vi "nanocal -- nuclear schottky fit -- 2x2 -- V9.vi"() -> ()   [LabVIEW 2021] (continued)
\"mm1\" -> 0.000000000000   ,  \"mm2\" -> 0.000000000000   ,  \"mm3\" -> 0.000000000000   ,  \"T\" -> 1.120000000000   ,  \"B\" -> 10.000000000000   ,  \"θ\" -> 0.000000000000   ,  \"Reoff\" -> 0.000000000000   ,  \"Imoff\" -> 0.000000000000   ,  \"στ1\" -> 0.000000000000   ,  \"στS\" -> 0.000000000000   ,  \"στN\" -> 0.000000000000    |>   , \r\"IDS0436_220527_RAW_cal__ref_\" ->   <|    \"ζ\" -> 0.020634042480   ,  \"τ1\" -> 0.020416898580   ,  \"τS\" -> 0.013006754143   ,  \"τN\" -> 0.000157221748   ,  \"τC\" -> 0.001868338850   ,  \"κ0\" -> 0.000000012250   ,  \"mm1\" -> 0.000033184482   ,  \"mm2\" -> 0.014698009084   ,  \"mm3\" -> 0.020989645793   ,  \"T\" -> 1.900000000000   ,  \"B\" -> 10.000000000000   ,  \"θ\" -> 0.000000000000   ,  \"Reoff\" -> -693877.551020413636   ,  \"Imoff\" -> 0.000000000000   ,  \"στ1\" -> 0.001009802597   ,  \"στS\" -> 0.000108538250   ,  \"στN\" -> 0.000005592624    |>   , \r\"IDS0436_220527_RAW_cal__sam_\" ->   <|    \"ζ\" -> 0.000000000000   ,  \"τ1\" -> 0.000000000000   ,  \"τS\" -> 0.000000000000   ,  \"τN\" -> 0.000000000000   ,  \"τC\" -> 0.000000000000   ,  \"κ0\" -> 0.000000000000   ,  \"mm1\" -> 0.000000000000   ,  \"mm2\" -> 0.000000000000   ,  \"mm3\" -> 0.000000000000   ,  \"T\" -> 1.900000000000   ,  \"B\" -> 10.000000000000   ,  \"θ\" -> 0.000000000000   ,  \"Reoff\" -> 0.000000000000   ,  \"Imoff\" -> 0.000000000000   ,  \"στ1\" -> 0.000000000000   ,  \"στS\" -> 0.000000000000   ,  \"στN\" -> 0.000000000000    |>   , \r\"IDS0437_220527_RAW_cal__ref_\" ->   <|    \"ζ\" -> 0.017700486500   ,  \"τ1\" -> 0.021195716861   ,  \"τS\" -> 0.009553240691   ,  \"τN\" -> 0.000096318625   ,  \"τC\" -> 0.001777778444   ,  \"κ0\" -> 0.000000022000   ,  \"mm1\" -> 0.000026199986   ,  \"mm2\" -> 0.011360732885   ,  \"mm3\" -> 0.021406923644   ,  \"T\" -> 3.100000000000   ,  \"B\" -> 10.000000000000   ,  \"θ\" -> 0.000000000000   ,  \"Reoff\" -> -326530.612244898453   ,  \"Imoff\" -> 0.000000000000   ,  \"στ1\" -> 0.003823035587   ,  \"στS\" -> 0.000080670014   ,  \"στN\" -> 0.000008312416    |>   , \r\"IDS0437_220527_RAW_cal__sam_\" ->   <|    \"ζ\" -> 0.000000000000   ,  \"τ1\" -> 0.000000000000   ,  \"τS\" -> 0.000000000000   ,  \"τN\" -> 0.000000000000   ,  \"τC\" -> 0.000000000000   ,  \"κ0\" -> 0.000000000000   ,  \"mm1\" -> 0.000000000000   ,  \"mm2\" -> 0.000000000000   ,  \"mm3\" -> 0.000000000000   ,  \"T\" -> 3.100000000000   ,  \"B\" -> 10.000000000000   ,  \"θ\" -> 0.000000000000   ,  \"Reoff\" -> 0.000000000000   ,  \"Imoff\" -> 0.000000000000   ,  \"στ1\" -> 0.000000000000   ,  \"στS\" -> 0.000000000000   ,  \"στN\" -> 0.000000000000    |>   , \r\"IDS0438_220527_RAW_cal__ref_\" ->   <|    \"ζ\" -> 0.017333863476   ,  \"τ1\" -> 0.021487771905   ,  \"τS\" -> 0.006060943357   ,  \"τN\" -> 0.000094743973   ,  \"τC\" -> 0.001680463551   ,  \"κ0\" -> 0.000000054800   ,  \"mm1\" -> 0.000022565233   ,  \"mm2\" -> 0.007769356044   ,  \"mm3\" -> 0.021638703353   ,  \"T\" -> 5.700000000000   ,  \"B\" -> 10.000000000000   ,  \"θ\" -> 0.000000000000   ,  \"Reoff\" -> -102040.816326530650   ,  \"Imoff\" -> 0.000000000000   ,  \"στ1\" -> 0.003634760564   ,  \"στS\" -> 0.000066823566   ,  \"στN\" -> 0.000004946508    |>   , \r\"IDS0438_220527_RAW_cal__sam_\" ->   <|    \"ζ\" -> 0.000000000000   ,  \"τ1\" -> 0.000000000000   ,  \"τS\" -> 0.000000000000   ,  \"τN\" -> 0.000000000000   ,  \"τC\" -> 0.000000000000   ,  \"κ0\" -> 0.000000000000   ,  \"mm1\" -> 0.000000000000   ,  \"mm2\" -> 0.000000000000   ,  \"mm3\" -> 0.000000000000   ,  \"T\" -> 5.700000000000   ,  \"B\" -> 10.000000000000   ,  \"θ\" -> 0.000000000000   ,  \"Reoff\" -> 0.000000000000   ,  \"Imoff\" -> 0.000000000000   ,  \"στ1\" -> 0.000000000000   ,  \"στS\" -> 0.000000000000   ,  \"στN\" -> 0.000000000000    |>   , \r\"IDS0439_220527_RAW_cal__ref_\" ->   <|    \"ζ\" -> 0.020515660719   ,  \"τ1\" -> 0.020182411708   ,  \"τS\" -> 0.016419895032   ,  \"τN\" -> 0.000240616919   ,  \"τC\" -> 0.002259910162   ,  \"κ0\" -> 0.000000008010   ,  \"mm1\" -> 0.000040116981   ,  \"mm2\" -> 0.017425178232   ,  \"mm3\" -> 0.021979340018   ,  \"T\" -> 1.280000000000   ,  \"B\" -> 10.000000000000   ,  \"θ\" -> 0.000000000000   ,  \"Reoff\" -> -693877.551020413636   ,  \"Imoff\" -> 0.000000000000   ,  \"στ1\" -> 0.001720696083   ,  \"στS\" -> 0.000105898596   ,  \"στN\" -> 0.000011441558    |>   , \r\"IDS0439_220527_RAW_cal__sam_\" ->   <|    \"ζ\" -> 0.000000000000   ,  \"τ1\" -> 0.000000000000   ,  \"τS\" -> 0.000000000000   ,  \"τN\" -> 0.000000000000   ,  \"τC\" -> 0.000000000000   ,  \"κ0\" -> 0.000000000000   ,  \"mm1\" -> 0.000000000000   ,  \"mm2\" -> 0.000000000000   ,  \"mm3\" -> 0.000000000000   ,  \"T\" -> 1.280000000000   ,  \"B\" -> 10.000000000000   ,  \"θ\" -> 0.000000000000   ,  \"Reoff\" -> 0.000000000000   ,  \"Imoff\" -> 0.000000000000   ,  \"στ1\" -> 0.000000000000   ,  \"στS\" -> 0.000000000000   ,  \"στN\" -> 0.000000000000    |>   , \r\"IDS0441_220527_RAW_cal__ref_\" ->   <|    \"ζ\" -> 0.211856799532   ,  \"τ1\" -> 0.173713031248   ,  \"τS\" -> 0.025047077219   ,  \"τN\" -> 0.022799850294   ,  \"τC\" -> 0.001119487792   ,  \"κ0\" -> 0.000000000820   ,  \"mm1\" -> 0.000189887587   ,  \"mm2\" -> 0.026344768969   ,  \"mm3\" -> 0.206281486927   ,  \"T\" -> 0.200000000000   ,  \"B\" -> 6.000000000000   ,  \"θ\" -> 0.000000000000   ,  \"Reoff\" -> -7510204.081632658840   ,  \"Imoff\" -> 0.000000000000   ,  \"στ1\" -> 0.033514341427   ,  \"στS\" -> 0.000356628888   ,  \"στN\" -> 0.003953255270    |>   , \r\"IDS0441_220527_RAW_cal__sam_\" ->   <|    \"ζ\" -> 0.000000000000   ,  \"τ1\" -> 0.000000000000   ,  \"τS\" -> 0.000000000000   ,  \"τN\" -> 0.000000000000   ,  \"τC\" -> 0.000000000000   ,  \"κ0\" -> 0.000000000000   ,  \"mm1\" -> 0.000000000000   ,  \"mm2\" -> 0.000000000000   ,  \"mm3\" -> 0.000000000000   ,  \"T\" -> 0.200000000000   ,  \"B\" -> 6.000000000000   ,  \"θ\" -> 0.000000000000   ,  \"Reoff\" -> 0.000000000000   ,  \"Imoff\" -> 0.000000000000   ,  \"στ1\" -> 0.000000000000   ,  \"στS\" -> 0.000000000000   ,  \"στN\" -> 0.000000000000    |>   , \r\"IDS0442_220528_RAW_cal__ref_\" ->   <|    \"ζ\" -> 0.627289985820   ,  \"τ1\" -> 0.239743496780   ,  \"τS\" -> 0.076926495749   ,  \"τN\" -> 0.159415903746   ,  \"τC\" -> 0.000763641667   ,  \"κ0\" -> 0.000000000435   ,  \"mm1\" -> 0.000293264880   ,  \"mm2\" -> 0.052650493650   ,  \"mm3\" -> 0.572160999840   ,  \"T\" -> 0.120000000000   ,  \"B\" -> 6.000000000000   ,  \"θ\" -> 0.000000000000   ,  \"Reoff\" -> -187755102.040816367000   ,  \"Imoff\" -> 0.000000000000   ,  \"στ1\" -> 0.245568364347   ,  \"στS\" -> 0.022170590915   ,  \"στN\" -> 0.126655465898    |>   , \r\"IDS0442_220528_RAW_cal__sam_\" ->   <|    \"ζ\" -> 0.000000000000   ,  \"τ1\" -> 0.000000000000   ,  \"τS\" -> 0.000000000000   ,  \"τN\" -> 0.000000000000   ,  \"τC\" -> 0.000000000000   ,  \"κ0\" -> 0.000000000000   ,  \"mm1\" -> 0.000000000000   ,  \"mm2\" -> 0.000000000000   ,  \"mm3\" -> 0.000000000000   ,  \"T\" -> 0.120000000000   ,  \"B\" -> 6.000000000000   ,  \"θ\" -> 0.000000000000   ,  \"Reoff\" -> 0.000000000000   ,  \"Imoff\" -> 0.000000000000   ,  \"στ1\" -> 0.000000000000   ,  \"στS\" -> 0.000000000000   ,  \"στN\" -> 0.000000000000    |>   , \r\"IDS0443_220528_RAW_cal__ref_\" ->   <|    \"ζ\" -> 0.436035823116   ,  \"τ1\" -> 0.136298324856   ,  \"τS\" -> 0.035428802447   ,  \"τN\" -> 0.042141009445   ,  \"τC\" -> 0.000863434496   ,  \"κ0\" -> 0.000000000631   ,  \"mm1\" -> 0.000259087412   ,  \"mm2\" -> 0.032519927017   ,  \"mm3\" -> 0.215775773592   ,  \"T\" -> 0.150000000000   ,  \"B\" -> 6.000000000000   ,  \"θ\" -> 0.000000000000   ,  \"Reoff\" -> -60040816.326530613000   ,  \"Imoff\" -> 0.000000000000   ,  \"στ1\" -> 0.080047050506   ,  \"στS\" -> 0.002312030387   ,  \"στN\" -> 0.019370507574    |>   , \r\"IDS0443_220528_RAW_cal__sam_\" ->   <|    \"ζ\" -> 0.000000000000   ,  \"τ1\" -> 0.000000000000   ,  \"τS\" -> 0.000000000000   ,  \"τN\" -> 0.000000000000   ,  \"τC\" -> 0.000000000000   ,  \"κ0\" -> 0.000000000000   ,  \"mm1\" -> 0.000000000000   ,  \"mm2\" -> 0.000000000000   ,  \"mm3\" -> 0.000000000000   ,  \"T\" -> 0.150000000000   ,  \"B\" -> 6.000000000000   ,  \"θ\" -> 0.000000000000   ,  \"Reoff\" -> 0.000000000000   ,  \"Imoff\" -> 0.000000000000   ,  \"στ1\" -> 0.000000000000   ,  \"στS\" -> 0.000000000000   ,  \"στN\" -> 0.000000000000    |>   , \r\"IDS0444_220528_RAW_cal__ref_\" ->   <|    \"ζ\" -> 0.312738827075   ,  \"τ1\" -> 0.153166775684   ,  \"τS\" -> 0.029428403772   ,  \"τN\" -> 0.032059842595   ,  \"τC\" -> 0.000966119229   ,  \"κ0\" -> 0.000000000763   ,  \"mm1\" -> 0.000225827852   ,  \"mm2\" -> 0.029383297615   ,  \"mm3\" -> 0.205241777861   ,  \"T\" -> 0.170000000000   ,  \"B\" -> 6.000000000000   ,  \"θ\" -> 0.000000000000   ,  \"Reoff\" -> -20979591.836734697200   ,  \"Imoff\" -> 0.000000000000   ,  \"στ1\" -> 0.194871487206   ,  \"στS\" -> 0.001481931895   ,  \"στN\" -> 0.032515587695    |>   , \r\"IDS0444_220528_RAW_cal__sam_\" ->   <|    \"ζ\" -> 0.000000000000   ,  \"τ1\" -> 0.000000000000   ,  \"τS\" -> 0.000000000000   ,  \"τN\" -> 0.000000000000   ,  \"τC\" -> 0.000000000000   ,  \"κ0\" -> 0.000000000000   ,  \"mm1\" -> 0.000000000000   ,  \"mm2\" -> 0.000000000000   ,  \"mm3\" -> 0.000000000000   ,  \"T\" -> 0.170000000000   ,  \"B\" -> 6.000000000000   ,  \"θ\" -> 0.000000000000   ,  \"Reoff\" -> 0.000000000000   ,  \"Imoff\" -> 0.000000000000   ,  \"στ1\" -> 0.000000000000   ,  \"στS\" -> 0.000000000000   ,  \"στN\" -> 0.000000000000    |>   , \r\"IDS0445_220528_RAW_cal__ref_\" ->   <|    \"ζ\" -> 0.144974292956   ,  \"τ1\" -> 0.278153679109   ,  \"τS\" -> 0.020087180736   ,  \"τN\" -> 0.018878235169   ,  \"τC\" -> 0.001360650262   ,  \"κ0\" -> 0.000000001251   ,  \"mm1\" -> 0.000163756081   ,  \"mm2\" -> 0.022311875645   ,  \"mm3\" -> 0.301653097172   ,  \"T\" -> 0.250000000000   ,  \"B\" -> 6.000000000000   ,  \"θ\" -> 0.000000000000   ,  \"Reoff\" -> -857142.857142856343   ,  \"Imoff\" -> 0.000000000000   ,  \"στ1\" -> 0.021844314170   ,  \"στS\" -> 0.000158941721   ,  \"στN\" -> 0.001374609128    |>   , \r\"IDS0445_220528_RAW_cal__sam_\" ->   <|    \"ζ\" -> 0.000000000000   ,  \"τ1\" -> 0.000000000000   ,  \"τS\" -> 0.000000000000   ,  \"τN\" -> 0.000000000000   ,  \"τC\" -> 0.000000000000   ,  \"κ0\" -> 0.000000000000   ,  \"mm1\" -> 0.000000000000   ,  \"mm2\" -> 0.000000000000   ,  \"mm3\" -> 0.000000000000   ,  \"T\" -> 0.250000000000   ,  \"B\" -> 6.000000000000   ,  \"θ\" -> 0.000000000000   ,  \"Reoff\" -> 0.000000000000   ,  \"Imoff\" -> 0.000000000000   ,  \"στ1\" -> 0.000000000000   ,  \"στS\" -> 0.000000000000   ,  \"στN\" -> 0.000000000000    |>   , \r\"IDS0446_220528_RAW_cal__ref_\" ->   <|    \"ζ\" -> 0.103205072553   ,  \"τ1\" -> 0.456877167810   ,  \"τS\" -> 0.018190810680   ,  \"τN\" -> 0.020353539569   ,  \"τC\" -> 0.001532633678   ,  \"κ0\" -> 0.000000001557   ,  \"mm1\" -> 0.000134033999   ,  \"mm2\" -> 0.020416907251   ,  \"mm3\" -> 0.480381182951   ,  \"T\" -> 0.300000000000   ,  \"B\" -> 6.000000000000   ,  \"θ\" -> 0.000000000000   ,  \"Reoff\" -> -461224.489795918343   ,  \"Imoff\" -> 0.000000000000   ,  \"στ1\" -> 0.032347659490   ,  \"στS\" -> 0.000102258041   ,  \"στN\" -> 0.001172701872    |>   , \r\"IDS0446_220528_RAW_cal__sam_\" ->   <|    \"ζ\" -> 0.000000000000   ,  \"τ1\" -> 0.000000000000   ,  \"τS\" -> 0.000000000000   ,  \"τN\" -> 0.000000000000   ,  \"τC\" -> 0.000000000000   ,  \"κ0\" -> 0.000000000000   ,  \"mm1\" -> 0.000000000000   ,  \"mm2\" -> 0.000000000000   ,  \"mm3\" -> 0.000000000000   ,  \"T\" -> 0.300000000000   ,  \"B\" -> 6.000000000000   ,  \"θ\" -> 0.000000000000   ,  \"Reoff\" -> 0.000000000000   ,  \"Imoff\" -> 0.000000000000   ,  \"στ1\" -> 0.000000000000   ,  \"στS\" -> 0.000000000000   ,  \"στN\" -> 0.000000000000    |>   , \r\"IDS0447_220528_RAW_cal__ref_\" ->   <|    \"ζ\" -> 0.067386498273   ,  \"τ1\" -> 0.033759383158   ,  \"τS\" -> 0.016352467508   ,  \"τN\" -> 0.000055602042   ,  \"τC\" -> 0.002052818742   ,  \"κ0\" -> 0.000000002053   ,  \"mm1\" -> 0.000116658355   ,  \"mm2\" -> 0.019311291178   ,  \"mm3\" -> 0.033898004267   ,  \"T\" -> 0.360000000000   ,  \"B\" -> 6.000000000000   ,  \"θ\" -> 0.000000000000   ,  \"Reoff\" -> 4122448.979591837150   ,  \"Imoff\" -> 0.000000000000   ,  \"στ1\" -> 0.002480419110   ,  \"στS\" -> 0.000128292028   ,  \"στN\" -> 0.000001339614    |>   , \r\"IDS0447_220528_RAW_cal__sam_\" ->   <|    \"ζ\" -> 0.000000000000   ,  \"τ1\" -> 0.000000000000   ,  \"τS\" -> 0.000000000000   ,  \"τN\" -> 0.000000000000   ,  \"τC\" -> 0.000000000000   ,  \"κ0\" -> 0.000000000000   ,  \"mm1\" -> 0.000000000000   ,  \"mm2\" -> 0.000000000000   ,  \"mm3\" -> 0.000000000000   ,  \"T\" -> 0.360000000000   ,  \"B\" -> 6.000000000000   ,  \"θ\" -> 0.000000000000   ,  \"Reoff\" -> 0.000000000000   ,  \"Imoff\" -> 0.000000000000   ,  \"στ1\" -> 0.000000000000   ,  \"στS\" -> 0.000000000000   ,  \"στN\" -> 0.000000000000    |>   , \r\"IDS0448_220528_RAW_cal__ref_\" ->   <|    \"ζ\" -> 0.022507492936   ,  \"τ1\" -> 0.033871434243   ,  \"τS\" -> 0.016835987173   ,  \"τN\" -> 0.000213468402   ,  \"τC\" -> 0.001778165835   ,  \"κ0\" -> 0.000000002480   ,  \"mm1\" -> 0.000035543102   ,  \"mm2\" -> 0.018688914469   ,  \"mm3\" -> 0.034358338584   ,  \"T\" -> 0.420000000000   ,  \"B\" -> 6.000000000000   ,  \"θ\" -> 0.000000000000   ,  \"Reoff\" -> 4122448.979591837150   ,  \"Imoff\" -> 0.000000000000   ,  \"στ1\" -> 0.007814821926   ,  \"στS\" -> 0.000385740474   ,  \"στN\" -> 0.000018309382    |>   , \r\"IDS0448_220528_RAW_cal__sam_\" ->   <|    \"ζ\" -> 0.000000000000   ,  \"τ1\" -> 0.000000000000   ,  \"τS\" -> 0.000000000000   ,  \"τN\" -> 0.000000000000   ,  \"τC\" -> 0.000000000000   ,  \"κ0\" -> 0.000000000000   ,  \"mm1\" -> 0.000000000000   ,  \"mm2\" -> 0.000000000000   ,  \"mm3\" -> 0.000000000000   ,  \"T\" -> 0.420000000000   ,  \"B\" -> 6.000000000000   ,  \"θ\" -> 0.000000000000   ,  \"Reoff\" -> 0.000000000000   ,  \"Imoff\" -> 0.000000000000   ,  \"στ1\" -> 0.000000000000   ,  \"στS\" -> 0.000000000000   ,  \"στN\" -> 0.000000000000    |>   , \r\"IDS0449_220528_RAW_cal__ref_\" ->   <|    \"ζ\" -> 0.021849716435   ,  \"τ1\" -> 0.033883152649   ,  \"τS\" -> 0.018197027738   ,  \"τN\" -> 0.000213402501   ,  \"τC\" -> 0.001801850307   ,  \"κ0\" -> 0.000000003131   ,  \"mm1\" -> 0.000035185130   ,  \"mm2\" -> 0.020045453610   ,  \"mm3\" -> 0.034417057136   ,  \"T\" -> 0.520000000000   ,  \"B\" -> 6.000000000000   ,  \"θ\" -> 0.000000000000   ,  \"Reoff\" -> 4122448.979591837150   ,  \"Imoff\" -> 0.000000000000   ,  \"στ1\" -> 0.005200135882   ,  \"στS\" -> 0.000196781752   ,  \"στN\" -> 0.000016694885    |>   , \r\"IDS0449_220528_RAW_cal__sam_\" ->   <|    \"ζ\" -> 0.000000000000   ,  \"τ1\" -> 0.000000000000   ,  \"τS\" -> 0.000000000000   ,  \"τN\" -> 0.000000000000   ,  \"τC\" -> 0.000000000000   ,  \"κ0\" -> 0.000000000000   ,  \"mm1\" -> 0.000000000000   ,  \"mm2\" -> 0.000000000000   ,  \"mm3\" -> 0.000000000000   ,  \"T\" -> 0.520000000000   ,  \"B\" -> 6.000000000000   ,  \"θ\" -> 0.000000000000   ,  \"Reoff\" -> 0.000000000000   ,  \"Imoff\" -> 0.000000000000   ,  \"στ1\" -> 0.000000000000   ,  \"στS\" -> 0.000000000000   ,  \"στN\" -> 0.000000000000    |>   , \r\"IDS0450_220528_RAW_cal__ref_\" ->   <|    \"ζ\" -> 0.021729475893   ,  \"τ1\" -> 0.033901786343   ,  \"τS\" -> 0.020153498516   ,  \"τN\" -> 0.000213217921   ,  \"τC\" -> 0.001808973424   ,  \"κ0\" -> 0.000000003806   ,  \"mm1\" -> 0.000035421184   ,  \"mm2\" -> 0.021964202896   ,  \"mm3\" -> 0.034520410198   ,  \"T\" -> 0.620000000000   ,  \"B\" -> 6.000000000000   ,  \"θ\" -> 0.000000000000   ,  \"Reoff\" -> 3061224.489795919510   ,  \"Imoff\" -> 0.000000000000   ,  \"στ1\" -> 0.006296094438   ,  \"στS\" -> 0.000269248074   ,  \"στN\" -> 0.000016264647    |>   , \r\"IDS0450_220528_RAW_cal__sam_\" ->   <|    \"ζ\" -> 0.000000000000   ,  \"τ1\" -> 0.000000000000   ,  \"τS\" -> 0.000000000000   ,  \"τN\" -> 0.000000000000   ,  \"τC\" -> 0.000000000000   ,  \"κ0\" -> 0.000000000000   ,  \"mm1\" -> 0.000000000000   ,  \"mm2\" -> 0.000000000000   ,  \"mm3\" -> 0.000000000000   ,  \"T\" -> 0.620000000000   ,  \"B\" -> 6.000000000000   ,  \"θ\" -> 0.000000000000   ,  \"Reoff\" -> 0.000000000000   ,  \"Imoff\" -> 0.000000000000   ,  \"στ1\" -> 0.000000000000   ,  \"στS\" -> 0.000000000000   ,  \"στN\" -> 0.000000000000    |>   , \r\"IDS0451_220528_RAW_cal__ref_\" ->   <|    \"ζ\" -> 0.019851972634   ,  \"τ1\" -> 0.033846561532   ,  \"τS\" -> 0.023547995636   ,  \"τN\" -> 0.000274131753   ,  \"τC\" -> 0.002984103948   ,  \"κ0\" -> 0.000000005214   ,  \"mm1\" -> 0.000051766319   ,  \"mm2\" -> 0.026018760545   ,  \"mm3\" -> 0.035055182225   ,  \"T\" -> 0.820000000000   ,  \"B\" -> 6.000000000000   ,  \"θ\" -> 0.000000000000   ,  \"Reoff\" -> 40816.326530613005   ,  \"Imoff\" -> 0.000000000000   ,  \"στ1\" -> 0.001908169809   ,  \"στS\" -> 0.000133930876   ,  \"στN\" -> 0.000002638452    |>   , \r\"IDS0451_220528_RAW_cal__sam_\" ->   <|    \"ζ\" -> 0.000000000000   ,  \"τ1\" -> 0.000000000000   ,  \"τS\" -> 0.000000000000   ,  \"τN\" -> 0.000000000000   ,  \"τC\" -> 0.000000000000   ,  \"κ0\" -> 0.000000000000   ,  \"mm1\" -> 0.000000000000   ,  \"mm2\" -> 0.000000000000   ,  \"mm3\" -> 0.000000000000   ,  \"T\" -> 0.820000000000   ,  \"B\" -> 6.000000000000   ,  \"θ\" -> 0.000000000000   ,  \"Reoff\" -> 0.000000000000   ,  \"Imoff\" -> 0.000000000000   ,  \"στ1\" -> 0.000000000000   ,  \"στS\" -> 0.000000000000   ,  \"στN\" -> 0.000000000000    |>   , \r\"IDS0452_220528_RAW_cal__ref_\" ->   <|    \"ζ\" -> 0.016283381951   ,  \"τ1\" -> 0.033904524460   ,  \"τS\" -> 0.031661688913   ,  \"τN\" -> 0.000274537016   ,  \"τC\" -> 0.003250738485   ,  \"κ0\" -> 0.000000007263   ,  \"mm1\" -> 0.000047369067   ,  \"mm2\" -> 0.031583889293   ,  \"mm3\" -> 0.037980260279   ,  \"T\" -> 1.120000000000   ,  \"B\" -> 6.000000000000   ,  \"θ\" -> 0.000000000000   ,  \"Reoff\" -> 40816.326530613005   ,  \"Imoff\" -> 0.000000000000   ,  \"στ1\" -> 0.002257620140   ,  \"στS\" -> 0.000162839807   ,  \"στN\" -> 0.000009699550    |>   , \r\"IDS0452_220528_RAW_cal__sam_\" ->   <|    \"ζ\" -> 0.000000000000   ,  \"τ1\" -> 0.000000000000   ,  \"τS\" -> 0.000000000000   ,  \"τN\" -> 0.000000000000   ,  \"τC\" -> 0.000000000000   ,  \"κ0\" -> 0.000000000000   ,  \"mm1\" -> 0.000000000000   ,  \"mm2\" -> 0.000000000000   ,  \"mm3\" -> 0.000000000000   ,  \"T\" -> 1.120000000000   ,  \"B\" -> 6.000000000000   ,  \"θ\" -> 0.000000000000   ,  \"Reoff\" -> 0.000000000000   ,  \"Imoff\" -> 0.000000000000   ,  \"στ1\" -> 0.000000000000   ,  \"στS\" -> 0.000000000000   ,  \"στN\" -> 0.000000000000    |>   , \r\"IDS0453_220529_RAW_cal__ref_\" ->   <|    \"ζ\" -> 0.018860897000   ,  \"τ1\" -> 0.033783692310   ,  \"τS\" -> 0.033495916545   ,  \"τN\" -> 0.000426157498   ,  \"τC\" -> 0.003160296043   ,  \"κ0\" -> 0.000000011406   ,  \"mm1\" -> 0.000053621310   ,  \"mm2\" -> 0.031431982647   ,  \"mm3\" -> 0.040020259184   ,  \"T\" -> 1.700000000000   ,  \"B\" -> 6.000000000000   ,  \"θ\" -> 0.000000000000   ,  \"Reoff\" -> -371428.571428571827   ,  \"Imoff\" -> 0.000000000000   ,  \"στ1\" -> 0.008605835969   ,  \"στS\" -> 0.000457782614   ,  \"στN\" -> 0.000070271904    |>   , \r\"IDS0453_220529_RAW_cal__sam_\" ->   <|    \"ζ\" -> 0.000000000000   ,  \"τ1\" -> 0.000000000000   ,  \"τS\" -> 0.000000000000   ,  \"τN\" -> 0.000000000000   ,  \"τC\" -> 0.000000000000   ,  \"κ0\" -> 0.000000000000   ,  \"mm1\" -> 0.000000000000   ,  \"mm2\" -> 0.000000000000   ,  \"mm3\" -> 0.000000000000   ,  \"T\" -> 1.700000000000   ,  \"B\" -> 6.000000000000   ,  \"θ\" -> 0.000000000000   ,  \"Reoff\" -> 0.000000000000   ,  \"Imoff\" -> 0.000000000000   ,  \"στ1\" -> 0.000000000000   ,  \"στS\" -> 0.000000000000   ,  \"στN\" -> 0.000000000000    |>   , \r\"IDS0454_220529_RAW_cal__ref_\" ->   <|    \"ζ\" -> 0.017534515106   ,  \"τ1\" -> 0.023238617838   ,  \"τS\" -> 0.014265591932   ,  \"τN\" -> 0.000383027801   ,  \"τC\" -> 0.002949269667   ,  \"κ0\" -> 0.000000012895   ,  \"mm1\" -> 0.000042342847   ,  \"mm2\" -> 0.016473998003   ,  \"mm3\" -> 0.024577022833   ,  \"T\" -> 1.900000000000   ,  \"B\" -> 6.000000000000   ,  \"θ\" -> 0.000000000000   ,  \"Reoff\" -> -371428.571428571827   ,  \"Imoff\" -> 0.000000000000   ,  \"στ1\" -> 0.002498996258   ,  \"στS\" -> 0.000312031837   ,  \"στN\" -> 0.000009499626    |>   , \r\"IDS0454_220529_RAW_cal__sam_\" ->   <|    \"ζ\" -> 0.000000000000   ,  \"τ1\" -> 0.000000000000   ,  \"τS\" -> 0.000000000000   ,  \"τN\" -> 0.000000000000   ,  \"τC\" -> 0.000000000000   ,  \"κ0\" -> 0.000000000000   ,  \"mm1\" -> 0.000000000000   ,  \"mm2\" -> 0.000000000000   ,  \"mm3\" -> 0.000000000000   ,  \"T\" -> 1.900000000000   ,  \"B\" -> 6.000000000000   ,  \"θ\" -> 0.000000000000   ,  \"Reoff\" -> 0.000000000000   ,  \"Imoff\" -> 0.000000000000   ,  \"στ1\" -> 0.000000000000   ,  \"στS\" -> 0.000000000000   ,  \"στN\" -> 0.000000000000    |>   , \r\"IDS0455_220529_RAW_cal__ref_\" ->   <|    \"ζ\" -> 0.016579016475   ,  \"τ1\" -> 0.029207680039   ,  \"τS\" -> 0.009191722708   ,  \"τN\" -> 0.000282214156   ,  \"τC\" -> 0.002421267657   ,  \"κ0\" -> 0.000000022277   ,  \"mm1\" -> 0.000031445020   ,  \"mm2\" -> 0.011546501346   ,  \"mm3\" -> 0.029682006750   ,  \"T\" -> 3.100000000000   ,  \"B\" -> 6.000000000000   ,  \"θ\" -> 0.000000000000   ,  \"Reoff\" -> -224489.795918366871   ,  \"Imoff\" -> 0.000000000000   ,  \"στ1\" -> 0.003215464239   ,  \"στS\" -> 0.000088801730   ,  \"στN\" -> 0.000015299267    |>   , \r\"IDS0455_220529_RAW_cal__sam_\" ->   <|    \"ζ\" -> 0.000000000000   ,  \"τ1\" -> 0.000000000000   ,  \"τS\" -> 0.000000000000   ,  \"τN\" -> 0.000000000000   ,  \"τC\" -> 0.000000000000   ,  \"κ0\" -> 0.000000000000   ,  \"mm1\" -> 0.000000000000   ,  \"mm2\" -> 0.000000000000   ,  \"mm3\" -> 0.000000000000   ,  \"T\" -> 3.100000000000   ,  \"B\" -> 6.000000000000   ,  \"θ\" -> 0.000000000000   ,  \"Reoff\" -> 0.000000000000   ,  \"Imoff\" -> 0.000000000000   ,  \"στ1\" -> 0.000000000000   ,  \"στS\" -> 0.000000000000   ,  \"στN\" -> 0.000000000000    |>   , \r\"IDS0456_220529_RAW_cal__ref_\" ->   <|    \"ζ\" -> 0.017491792324   ,  \"τ1\" -> 0.025875515293   ,  \"τS\" -> 0.005854448604   ,  \"τN\" -> 0.000336782612   ,  \"τC\" -> 0.002022629565   ,  \"κ0\" -> 0.000000054778   ,  \"mm1\" -> 0.000026042057   ,  \"mm2\" -> 0.007805583534   ,  \"mm3\" -> 0.026366046213   ,  \"T\" -> 5.700000000000   ,  \"B\" -> 6.000000000000   ,  \"θ\" -> 0.000000000000   ,  \"Reoff\" -> -77551.020408162847   ,  \"Imoff\" -> 0.000000000000   ,  \"στ1\" -> 0.003570816055   ,  \"στS\" -> 0.000072912365   ,  \"στN\" -> 0.000023576375    |>   , \r\"IDS0456_220529_RAW_cal__sam_\" ->   <|    \"ζ\" -> 0.000000000000   ,  \"τ1\" -> 0.000000000000   ,  \"τS\" -> 0.000000000000   ,  \"τN\" -> 0.000000000000   ,  \"τC\" -> 0.000000000000   ,  \"κ0\" -> 0.000000000000   ,  \"mm1\" -> 0.000000000000   ,  \"mm2\" -> 0.000000000000   ,  \"mm3\" -> 0.000000000000   ,  \"T\" -> 5.700000000000   ,  \"B\" -> 6.000000000000   ,  \"θ\" -> 0.000000000000   ,  \"Reoff\" -> 0.000000000000   ,  \"Imoff\" -> 0.000000000000   ,  \"στ1\" -> 0.000000000000   ,  \"στS\" -> 0.000000000000   ,  \"στN\" -> 0.000000000000    |>   , \r\"IDS0458_220529_RAW_cal__ref_\" ->   <|    \"ζ\" -> 0.258233838884   ,  \"τ1\" -> 0.194823836197   ,  \"τS\" -> 0.017297068774   ,  \"τN\" -> 0.011336600616   ,  \"τC\" -> 0.000861022284   ,  \"κ0\" -> 0.000000000878   ,  \"mm1\" -> 0.000171280662   ,  \"mm2\" -> 0.020753326511   ,  \"mm3\" -> 0.210788103067   ,  \"T\" -> 0.200000000000   ,  \"B\" -> 4.000000000000   ,  \"θ\" -> 0.000000000000   ,  \"Reoff\" -> -40000000.000000000000   ,  \"Imoff\" -> 0.000000000000   ,  \"στ1\" -> 0.011784060995   ,  \"στS\" -> 0.000101210120   ,  \"στN\" -> 0.000651260820    |>   , \r\"IDS0458_220529_RAW_cal__sam_\" ->   <|    \"ζ\" -> 0.000000000000   ,  \"τ1\" -> 0.000000000000   ,  \"τS\" -> 0.000000000000   ,  \"τN\" -> 0.000000000000   ,  \"τC\" -> 0.000000000000   ,  \"κ0\" -> 0.000000000000   ,  \"mm1\" -> 0.000000000000   ,  \"mm2\" -> 0.000000000000   ,  \"mm3\" -> 0.000000000000   ,  \"T\" -> 0.200000000000   ,  \"B\" -> 4.000000000000   ,  \"θ\" -> 0.000000000000   ,  \"Reoff\" -> 0.000000000000   ,  \"Imoff\" -> 0.000000000000   ,  \"στ1\" -> 0.000000000000   ,  \"στS\" -> 0.000000000000   ,  \"στN\" -> 0.000000000000    |>   , \r\"IDS0459_220529_RAW_cal__ref_\" ->   <|    \"ζ\" -> 0.141553441331   ,  \"τ1\" -> 0.275028685548   ,  \"τS\" -> 0.015047963076   ,  \"τN\" -> 0.008277224775   ,  \"τC\" -> 0.000952592092   ,  \"κ0\" -> 0.000000001241   ,  \"mm1\" -> 0.000112614213   ,  \"mm2\" -> 0.017380815596   ,  \"mm3\" -> 0.285114796291   ,  \"T\" -> 0.250000000000   ,  \"B\" -> 4.000000000000   ,  \"θ\" -> 0.000000000000   ,  \"Reoff\" -> -3469387.755102038380   ,  \"Imoff\" -> 0.000000000000   ,  \"στ1\" -> 0.080083912968   ,  \"στS\" -> 0.000323805497   ,  \"στN\" -> 0.002416154276    |>   , \r\"IDS0459_220529_RAW_cal__sam_\" ->   <|    \"ζ\" -> 0.000000000000   ,  \"τ1\" -> 0.000000000000   ,  \"τS\" -> 0.000000000000   ,  \"τN\" -> 0.000000000000   ,  \"τC\" -> 0.000000000000   ,  \"κ0\" -> 0.000000000000   ,  \"mm1\" -> 0.000000000000   ,  \"mm2\" -> 0.000000000000   ,  \"mm3\" -> 0.000000000000   ,  \"T\" -> 0.250000000000   ,  \"B\" -> 4.000000000000   ,  \"θ\" -> 0.000000000000   ,  \"Reoff\" -> 0.000000000000   ,  \"Imoff\" -> 0.000000000000   ,  \"στ1\" -> 0.000000000000   ,  \"στS\" -> 0.000000000000   ,  \"στN\" -> 0.000000000000    |>   , \r\"IDS0460_220529_RAW_cal__ref_\" ->   <|    \"ζ\" -> 0.100306525535   ,  \"τ1\" -> 0.323446583464   ,  \"τS\" -> 0.014112138770   ,  \"τN\" -> 0.006689862663   ,  \"τC\" -> 0.001003931407   ,  \"κ0\" -> 0.000000001578   ,  \"mm1\" -> 0.000086413968   ,  \"mm2\" -> 0.016060715827   ,  \"mm3\" -> 0.331191962998   ,  \"T\" -> 0.300000000000   ,  \"B\" -> 4.000000000000   ,  \"θ\" -> 0.000000000000   ,  \"Reoff\" -> -1346938.775510203090   ,  \"Imoff\" -> 0.000000000000   ,  \"στ1\" -> 0.228013917636   ,  \"στS\" -> 0.000228957843   ,  \"στN\" -> 0.004274163524    |>   , \r\"IDS0460_220529_RAW_cal__sam_\" ->   <|    \"ζ\" -> 0.000000000000   ,  \"τ1\" -> 0.000000000000   ,  \"τS\" -> 0.000000000000   ,  \"τN\" -> 0.000000000000   ,  \"τC\" -> 0.000000000000   ,  \"κ0\" -> 0.000000000000   ,  \"mm1\" -> 0.000000000000   ,  \"mm2\" -> 0.000000000000   ,  \"mm3\" -> 0.000000000000   ,  \"T\" -> 0.300000000000   ,  \"B\" -> 4.000000000000   ,  \"θ\" -> 0.000000000000   ,  \"Reoff\" -> 0.000000000000   ,  \"Imoff\" -> 0.000000000000   ,  \"στ1\" -> 0.000000000000   ,  \"στS\" -> 0.000000000000   ,  \"στN\" -> 0.000000000000    |>   , \r\"IDS0461_220529_RAW_cal__ref_\" ->   <|    \"ζ\" -> 0.071863540355   ,  \"τ1\" -> 0.372398952116   ,  \"τS\" -> 0.013146723142   ,  \"τN\" -> 0.005489502105   ,  \"τC\" -> 0.001555491237   ,  \"κ0\" -> 0.000000001966   ,  \"mm1\" -> 0.000094490759   ,  \"mm2\" -> 0.015300544387   ,  \"mm3\" -> 0.378534898581   ,  \"T\" -> 0.360000000000   ,  \"B\" -> 4.000000000000   ,  \"θ\" -> 0.000000000000   ,  \"Reoff\" -> 40816.326530613005   ,  \"Imoff\" -> 0.000000000000   ,  \"στ1\" -> 0.066981077453   ,  \"στS\" -> 0.000100786284   ,  \"στN\" -> 0.000881671068    |>   , \r\"IDS0461_220529_RAW_cal__sam_\" ->   <|    \"ζ\" -> 0.000000000000   ,  \"τ1\" -> 0.000000000000   ,  \"τS\" -> 0.000000000000   ,  \"τN\" -> 0.000000000000   ,  \"τC\" -> 0.000000000000   ,  \"κ0\" -> 0.000000000000   ,  \"mm1\" -> 0.000000000000   ,  \"mm2\" -> 0.000000000000   ,  \"mm3\" -> 0.000000000000   ,  \"T\" -> 0.360000000000   ,  \"B\" -> 4.000000000000   ,  \"θ\" -> 0.000000000000   ,  \"Reoff\" -> 0.000000000000   ,  \"Imoff\" -> 0.000000000000   ,  \"στ1\" -> 0.000000000000   ,  \"στS\" -> 0.000000000000   ,  \"στN\" -> 0.000000000000    |>   , \r\"IDS0462_220530_RAW_cal__ref_\" ->   <|    \"ζ\" -> 0.346375365864   ,  \"τ1\" -> 0.255981907492   ,  \"τS\" -> 0.020113199989   ,  \"τN\" -> 0.019024971264   ,  \"τC\" -> 0.000835805308   ,  \"κ0\" -> 0.000000000713   ,  \"mm1\" -> 0.000210164212   ,  \"mm2\" -> 0.024940973157   ,  \"mm3\" -> 0.284361245071   ,  \"T\" -> 0.170000000000   ,  \"B\" -> 4.000000000000   ,  \"θ\" -> 0.000000000000   ,  \"Reoff\" -> -62857142.857142865700   ,  \"Imoff\" -> 0.000000000000   ,  \"στ1\" -> 0.079526914499   ,  \"στS\" -> 0.000288042615   ,  \"στN\" -> 0.004319163627    |>   , \r\"IDS0462_220530_RAW_cal__sam_\" ->   <|    \"ζ\" -> 0.000000000000   ,  \"τ1\" -> 0.000000000000   ,  \"τS\" -> 0.000000000000   ,  \"τN\" -> 0.000000000000   ,  \"τC\" -> 0.000000000000   ,  \"κ0\" -> 0.000000000000   ,  \"mm1\" -> 0.000000000000   ,  \"mm2\" -> 0.000000000000   ,  \"mm3\" -> 0.000000000000   ,  \"T\" -> 0.170000000000   ,  \"B\" -> 4.000000000000   ,  \"θ\" -> 0.000000000000   ,  \"Reoff\" -> 0.000000000000   ,  \"Imoff\" -> 0.000000000000   ,  \"στ1\" -> 0.000000000000   ,  \"στS\" -> 0.000000000000   ,  \"στN\" -> 0.000000000000    |>   , \r\"IDS0463_220530_RAW_cal__ref_\" ->   <|    \"ζ\" -> 0.446275337285   ,  \"τ1\" -> 0.266780954732   ,  \"τS\" -> 0.022382001002   ,  \"τN\" -> 0.026082260900   ,  \"τC\" -> 0.000765140515   ,  \"κ0\" -> 0.000000000610   ,  \"mm1\" -> 0.000232271004   ,  \"mm2\" -> 0.028408418126   ,  \"mm3\" -> 0.308998072845   ,  \"T\" -> 0.150000000000   ,  \"B\" -> 4.000000000000   ,  \"θ\" -> 0.000000000000   ,  \"Reoff\" -> -99591836.734693884900   ,  \"Imoff\" -> 0.000000000000   ,  \"στ1\" -> 0.224882550084   ,  \"στS\" -> 0.000618191534   ,  \"στN\" -> 0.017485695172    |>   , \r\"IDS0463_220530_RAW_cal__sam_\" ->   <|    \"ζ\" -> 0.000000000000   ,  \"τ1\" -> 0.000000000000   ,  \"τS\" -> 0.000000000000   ,  \"τN\" -> 0.000000000000   ,  \"τC\" -> 0.000000000000   ,  \"κ0\" -> 0.000000000000   ,  \"mm1\" -> 0.000000000000   ,  \"mm2\" -> 0.000000000000   ,  \"mm3\" -> 0.000000000000   ,  \"T\" -> 0.150000000000   ,  \"B\" -> 4.000000000000   ,  \"θ\" -> 0.000000000000   ,  \"Reoff\" -> 0.000000000000   ,  \"Imoff\" -> 0.000000000000   ,  \"στ1\" -> 0.000000000000   ,  \"στS\" -> 0.000000000000   ,  \"στN\" -> 0.000000000000    |>   , \r\"IDS0464_220530_RAW_cal__ref_\" ->   <|    \"ζ\" -> 0.686294435706   ,  \"τ1\" -> 0.209764249284   ,  \"τS\" -> 0.029859376901   ,  \"τN\" -> 0.037449784740   ,  \"τC\" -> 0.000759618716   ,  \"κ0\" -> 0.000000000451   ,  \"mm1\" -> 0.000306389512   ,  \"mm2\" -> 0.037194660007   ,  \"mm3\" -> 0.286525883228   ,  \"T\" -> 0.120000000000   ,  \"B\" -> 4.000000000000   ,  \"θ\" -> 0.000000000000   ,  \"Reoff\" -> -184081632.653061211000   ,  \"Imoff\" -> 0.000000000000   ,  \"στ1\" -> 0.142338002900   ,  \"στS\" -> 0.001307467027   ,  \"στN\" -> 0.020432553126    |>   , \r\"IDS0464_220530_RAW_cal__sam_\" ->   <|    \"ζ\" -> 0.000000000000   ,  \"τ1\" -> 0.000000000000   ,  \"τS\" -> 0.000000000000   ,  \"τN\" -> 0.000000000000   ,  \"τC\" -> 0.000000000000   ,  \"κ0\" -> 0.000000000000   ,  \"mm1\" -> 0.000000000000   ,  \"mm2\" -> 0.000000000000   ,  \"mm3\" -> 0.000000000000   ,  \"T\" -> 0.120000000000   ,  \"B\" -> 4.000000000000   ,  \"θ\" -> 0.000000000000   ,  \"Reoff\" -> 0.000000000000   ,  \"Imoff\" -> 0.000000000000   ,  \"στ1\" -> 0.000000000000   ,  \"στS\" -> 0.000000000000   ,  \"στN\" -> 0.000000000000    |>   , \r\"IDS0465_220530_RAW_cal__ref_\" ->   <|    \"ζ\" -> 0.053585302265   ,  \"τ1\" -> 0.387212962243   ,  \"τS\" -> 0.013176914170   ,  \"τN\" -> 0.005324197472   ,  \"τC\" -> 0.001817109761   ,  \"κ0\" -> 0.000000002434   ,  \"mm1\" -> 0.000082150851   ,  \"mm2\" -> 0.015385999012   ,  \"mm3\" -> 0.393054421443   ,  \"T\" -> 0.430000000000   ,  \"B\" -> 4.000000000000   ,  \"θ\" -> 0.000000000000   ,  \"Reoff\" -> -40816.326530611142   ,  \"Imoff\" -> 0.000000000000   ,  \"στ1\" -> 0.094015182018   ,  \"στS\" -> 0.000095156235   ,  \"στN\" -> 0.001056636075    |>   , \r\"IDS0465_220530_RAW_cal__sam_\" ->   <|    \"ζ\" -> 0.000000000000   ,  \"τ1\" -> 0.000000000000   ,  \"τS\" -> 0.000000000000   ,  \"τN\" -> 0.000000000000   ,  \"τC\" -> 0.000000000000   ,  \"κ0\" -> 0.000000000000   ,  \"mm1\" -> 0.000000000000   ,  \"mm2\" -> 0.000000000000   ,  \"mm3\" -> 0.000000000000   ,  \"T\" -> 0.430000000000   ,  \"B\" -> 4.000000000000   ,  \"θ\" -> 0.000000000000   ,  \"Reoff\" -> 0.000000000000   ,  \"Imoff\" -> 0.000000000000   ,  \"στ1\" -> 0.000000000000   ,  \"στS\" -> 0.000000000000   ,  \"στN\" -> 0.000000000000    |>   , \r\"IDS0466_220530_RAW_cal__ref_\" ->   <|    \"ζ\" -> 0.040587802625   ,  \"τ1\" -> 0.301310985545   ,  \"τS\" -> 0.013808867786   ,  \"τN\" -> 0.003299045809   ,  \"τC\" -> 0.002151008658   ,  \"κ0\" -> 0.000000003055   ,  \"mm1\" -> 0.000073300109   ,  \"mm2\" -> 0.016251460699   ,  \"mm3\" -> 0.304939519611   ,  \"T\" -> 0.530000000000   ,  \"B\" -> 4.000000000000   ,  \"θ\" -> 0.000000000000   ,  \"Reoff\" -> -100000.000000000000   ,  \"Imoff\" -> 0.000000000000   ,  \"στ1\" -> 0.058870051351   ,  \"στS\" -> 0.000095860880   ,  \"στN\" -> 0.000149332879    |>   , \r\"IDS0466_220530_RAW_cal__sam_\" ->   <|    \"ζ\" -> 0.000000000000   ,  \"τ1\" -> 0.000000000000   ,  \"τS\" -> 0.000000000000   ,  \"τN\" -> 0.000000000000   ,  \"τC\" -> 0.000000000000   ,  \"κ0\" -> 0.000000000000   ,  \"mm1\" -> 0.000000000000   ,  \"mm2\" -> 0.000000000000   ,  \"mm3\" -> 0.000000000000   ,  \"T\" -> 0.530000000000   ,  \"B\" -> 4.000000000000   ,  \"θ\" -> 0.000000000000   ,  \"Reoff\" -> 0.000000000000   ,  \"Imoff\" -> 0.000000000000   ,  \"στ1\" -> 0.000000000000   ,  \"στS\" -> 0.000000000000   ,  \"στN\" -> 0.000000000000    |>   , \r\"IDS0467_220530_RAW_cal__ref_\" ->   <|    \"ζ\" -> 0.033721890656   ,  \"τ1\" -> 0.305158658126   ,  \"τS\" -> 0.015259706261   ,  \"τN\" -> 0.003270549232   ,  \"τC\" -> 0.002211339176   ,  \"κ0\" -> 0.000000003708   ,  \"mm1\" -> 0.000063492332   ,  \"mm2\" -> 0.017713895479   ,  \"mm3\" -> 0.308747740233   ,  \"T\" -> 0.620000000000   ,  \"B\" -> 4.000000000000   ,  \"θ\" -> 0.000000000000   ,  \"Reoff\" -> -530612.244897957890   ,  \"Imoff\" -> 0.000000000000   ,  \"στ1\" -> 0.037196884325   ,  \"στS\" -> 0.000076701632   ,  \"στN\" -> 0.000400525056    |>   , \r\"IDS0467_220530_RAW_cal__sam_\" ->   <|    \"ζ\" -> 0.000000000000   ,  \"τ1\" -> 0.000000000000   ,  \"τS\" -> 0.000000000000   ,  \"τN\" -> 0.000000000000   ,  \"τC\" -> 0.000000000000   ,  \"κ0\" -> 0.000000000000   ,  \"mm1\" -> 0.000000000000   ,  \"mm2\" -> 0.000000000000   ,  \"mm3\" -> 0.000000000000   ,  \"T\" -> 0.620000000000   ,  \"B\" -> 4.000000000000   ,  \"θ\" -> 0.000000000000   ,  \"Reoff\" -> 0.000000000000   ,  \"Imoff\" -> 0.000000000000   ,  \"στ1\" -> 0.000000000000   ,  \"στS\" -> 0.000000000000   ,  \"στN\" -> 0.000000000000    |>   , \r\"IDS0468_220530_RAW_cal__ref_\" ->   <|    \"ζ\" -> 0.026965567816   ,  \"τ1\" -> 0.311333130890   ,  \"τS\" -> 0.019058177307   ,  \"τN\" -> 0.001637032675   ,  \"τC\" -> 0.002479362989   ,  \"κ0\" -> 0.000000005077   ,  \"mm1\" -> 0.000057934269   ,  \"mm2\" -> 0.021866564676   ,  \"mm3\" -> 0.313141263006   ,  \"T\" -> 0.820000000000   ,  \"B\" -> 4.000000000000   ,  \"θ\" -> 0.000000000000   ,  \"Reoff\" -> -775510.204081632196   ,  \"Imoff\" -> 0.000000000000   ,  \"στ1\" -> 0.011514473145   ,  \"στS\" -> 0.000124420798   ,  \"στN\" -> 0.000031809613    |>   , \r\"IDS0468_220530_RAW_cal__sam_\" ->   <|    \"ζ\" -> 0.000000000000   ,  \"τ1\" -> 0.000000000000   ,  \"τS\" -> 0.000000000000   ,  \"τN\" -> 0.000000000000   ,  \"τC\" -> 0.000000000000   ,  \"κ0\" -> 0.000000000000   ,  \"mm1\" -> 0.000000000000   ,  \"mm2\" -> 0.000000000000   ,  \"mm3\" -> 0.000000000000   ,  \"T\" -> 0.820000000000   ,  \"B\" -> 4.000000000000   ,  \"θ\" -> 0.000000000000   ,  \"Reoff\" -> 0.000000000000   ,  \"Imoff\" -> 0.000000000000   ,  \"στ1\" -> 0.000000000000   ,  \"στS\" -> 0.000000000000   ,  \"στN\" -> 0.000000000000    |>   , \r\"IDS0469_220530_RAW_cal__ref_\" ->   <|    \"ζ\" -> 0.015711519160   ,  \"τ1\" -> 0.318730278460   ,  \"τS\" -> 0.028371053970   ,  \"τN\" -> 0.001582585159   ,  \"τC\" -> 0.002541343037   ,  \"κ0\" -> 0.000000007141   ,  \"mm1\" -> 0.000036166583   ,  \"mm2\" -> 0.031147898286   ,  \"mm3\" -> 0.320511812932   ,  \"T\" -> 1.120000000000   ,  \"B\" -> 4.000000000000   ,  \"θ\" -> 0.000000000000   ,  \"Reoff\" -> -122448.979591835290   ,  \"Imoff\" -> 0.000000000000   ,  \"στ1\" -> 0.017857928261   ,  \"στS\" -> 0.000289333463   ,  \"στN\" -> 0.000005286527    |>   , \r\"IDS0469_220530_RAW_cal__sam_\" ->   <|    \"ζ\" -> 0.000000000000   ,  \"τ1\" -> 0.000000000000   ,  \"τS\" -> 0.000000000000   ,  \"τN\" -> 0.000000000000   ,  \"τC\" -> 0.000000000000   ,  \"κ0\" -> 0.000000000000   ,  \"mm1\" -> 0.000000000000   ,  \"mm2\" -> 0.000000000000   ,  \"mm3\" -> 0.000000000000   ,  \"T\" -> 1.120000000000   ,  \"B\" -> 4.000000000000   ,  \"θ\" -> 0.000000000000   ,  \"Reoff\" -> 0.000000000000   ,  \"Imoff\" -> 0.000000000000   ,  \"στ1\" -> 0.000000000000   ,  \"στS\" -> 0.000000000000   ,  \"στN\" -> 0.000000000000    |>   , \r\"IDS0470_220530_RAW_cal__ref_\" ->   <|    \"ζ\" -> 0.015683435262   ,  \"τ1\" -> 0.093477306412   ,  \"τS\" -> 0.036382915051   ,  \"τN\" -> 0.001214958460   ,  \"τC\" -> 0.002412472739   ,  \"κ0\" -> 0.000000012824   ,  \"mm1\" -> 0.000034999821   ,  \"mm2\" -> 0.038468098598   ,  \"mm3\" -> 0.095574218059   ,  \"T\" -> 1.900000000000   ,  \"B\" -> 4.000000000000   ,  \"θ\" -> 0.000000000000   ,  \"Reoff\" -> -224489.795918366871   ,  \"Imoff\" -> 0.000000000000   ,  \"στ1\" -> 0.010189622060   ,  \"στS\" -> 0.000541087053   ,  \"στN\" -> 0.000035341522    |>   , \r\"IDS0470_220530_RAW_cal__sam_\" ->   <|    \"ζ\" -> 0.000000000000   ,  \"τ1\" -> 0.000000000000   ,  \"τS\" -> 0.000000000000   ,  \"τN\" -> 0.000000000000   ,  \"τC\" -> 0.000000000000   ,  \"κ0\" -> 0.000000000000   ,  \"mm1\" -> 0.000000000000   ,  \"mm2\" -> 0.000000000000   ,  \"mm3\" -> 0.000000000000   ,  \"T\" -> 1.900000000000   ,  \"B\" -> 4.000000000000   ,  \"θ\" -> 0.000000000000   ,  \"Reoff\" -> 0.000000000000   ,  \"Imoff\" -> 0.000000000000   ,  \"στ1\" -> 0.000000000000   ,  \"στS\" -> 0.000000000000   ,  \"στN\" -> 0.000000000000    |>   , \r\"IDS0471_220530_RAW_cal__ref_\" ->   <|    \"ζ\" -> 0.015530188750   ,  \"τ1\" -> 0.057492054043   ,  \"τS\" -> 0.011355043068   ,  \"τN\" -> 0.002034995182   ,  \"τC\" -> 0.003067612418   ,  \"κ0\" -> 0.000000015408   ,  \"mm1\" -> 0.000037148295   ,  \"mm2\" -> 0.013903152221   ,  \"mm3\" -> 0.060217354016   ,  \"T\" -> 2.300000000000   ,  \"B\" -> 4.000000000000   ,  \"θ\" -> 0.000000000000   ,  \"Reoff\" -> -224489.795918366871   ,  \"Imoff\" -> 0.000000000000   ,  \"στ1\" -> 0.007617043980   ,  \"στS\" -> 0.000107126758   ,  \"στN\" -> 0.000086071439    |>   , \r\"IDS0471_220530_RAW_cal__sam_\" ->   <|    \"ζ\" -> 0.000000000000   ,  \"τ1\" -> 0.000000000000   ,  \"τS\" -> 0.000000000000   ,  \"τN\" -> 0.000000000000   ,  \"τC\" -> 0.000000000000   ,  \"κ0\" -> 0.000000000000   ,  \"mm1\" -> 0.000000000000   ,  \"mm2\" -> 0.000000000000   ,  \"mm3\" -> 0.000000000000   ,  \"T\" -> 2.300000000000   ,  \"B\" -> 4.000000000000   ,  \"θ\" -> 0.000000000000   ,  \"Reoff\" -> 0.000000000000   ,  \"Imoff\" -> 0.000000000000   ,  \"στ1\" -> 0.000000000000   ,  \"στS\" -> 0.000000000000   ,  \"στN\" -> 0.000000000000    |>   , \r\"IDS0472_220530_RAW_cal__ref_\" ->   <|    \"ζ\" -> 0.020183384873   ,  \"τ1\" -> 0.125148338394   ,  \"τS\" -> 0.009086310836   ,  \"τN\" -> 0.001084318795   ,  \"τC\" -> 0.002862624150   ,  \"κ0\" -> 0.000000022333   ,  \"mm1\" -> 0.000043426508   ,  \"mm2\" -> 0.011972013696   ,  \"mm3\" -> 0.126371429704   ,  \"T\" -> 3.070000000000   ,  \"B\" -> 4.000000000000   ,  \"θ\" -> 0.000000000000   ,  \"Reoff\" -> -224489.795918366871   ,  \"Imoff\" -> 0.000000000000   ,  \"στ1\" -> 0.012710988374   ,  \"στS\" -> 0.000085184926   ,  \"στN\" -> 0.000054449866    |>   , \r\"IDS0472_220530_RAW_cal__sam_\" ->   <|    \"ζ\" -> 0.000000000000   ,  \"τ1\" -> 0.000000000000   ,  \"τS\" -> 0.000000000000   ,  \"τN\" -> 0.000000000000   ,  
